vi "7L17_perso.vi"() -> ()   [LabVIEW 2010]
panel:
  out "Ccpc init":dbl
  in  "cas vrai":dbl
  in  "cas faux":dbl
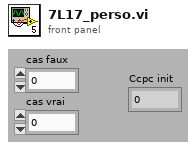
[diagram p1: front panel]
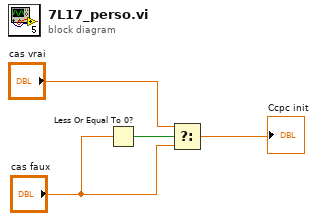
[diagram p0: block diagram]
diagram:
  n1 = Less Or Equal To 0?(x="cas faux") -> (x <= 0?=w4:bool)
  n2 = Select(t="cas vrai", s=w4, f="cas faux") -> (s? t:f=→"Ccpc init":dbl)
